vi "TX ADU.vi"(8 "error in (no error)":errorcluster, 9 "PDU_req in":T1={"Function Code"=1, "Data"=[], "RTU_DataBytes"=0}, 10 "VISA resource in":refnum<visa-resource-name>, 11 "MB_ADU in":refnum<class "MB_ADU_ASCII.lvclass">) -> (0 "error out":errorcluster, 1 "PDU_req out":T1={"Function Code"=1, "Data"=[], "RTU_DataBytes"=0}, 2 "VISA resource out":refnum<visa-resource-name>, 3 "MB_ADU out":refnum<class "MB_ADU_ASCII.lvclass">)   [LabVIEW 2012, in "MB Master.lvlib" / "MB_ADU_ASCII.lvclass"]
doc: "Defines the transmit procedure for a Modbus ASCII ADU. The PDU to be transmitted should be written to PDU_req prior to calling this VI."
uses:
  MB_ADU_ASCII.lvclass
  MB_PDU/MB_PDU_Cluster.ctl
  MB_ADU/MB_ADU.lvclass/MB_ADU.ctl
  MB_ADU/Read Slave ID.vi
  MB_ADU/Write TX Data.vi
  MB_ADU/Write TX Timestamp.vi
  MB Master.lvlib
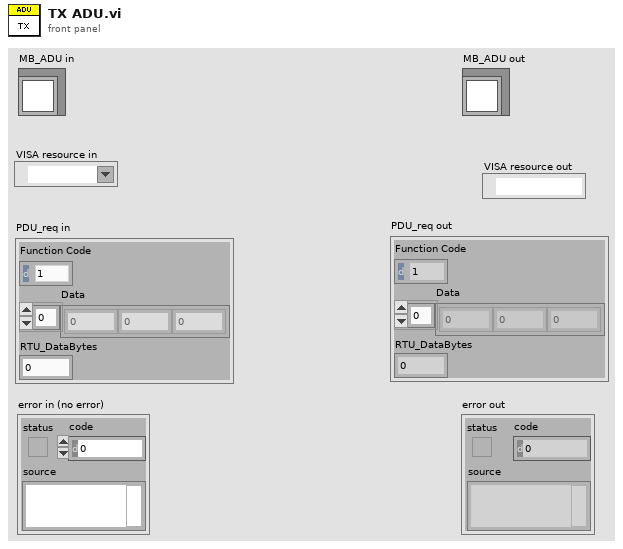
[diagram p1: front panel]
types:
  T1 = typedef "MB Master.lvlib/MB_PDU_Cluster.ctl" = cluster{"Function Code":u8, "Data":u8[], "RTU_DataBytes":i32}
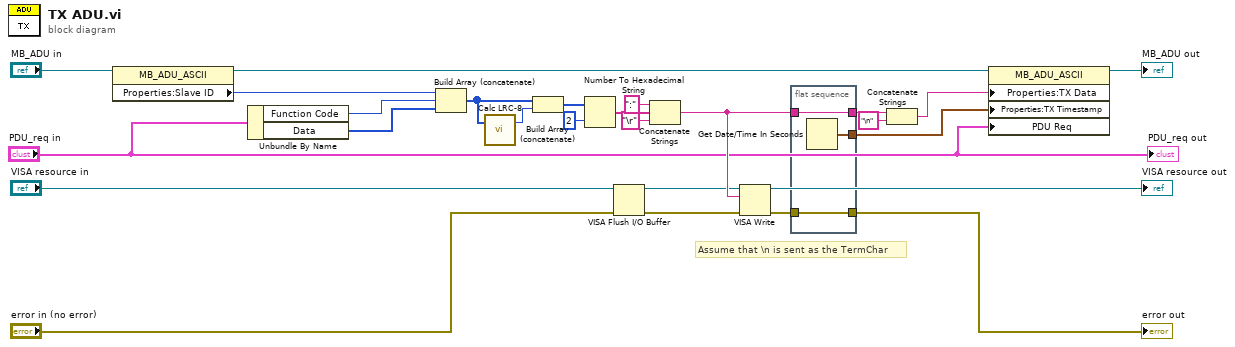
[diagram p0: block diagram]
diagram:
  # "Assume that \\n is sent as the TermChar"
  n1 = property class="MB_ADU_ASCII"(reference="MB_ADU in") -> (reference out=w11:refnum<class "MB_ADU_ASCII.lvclass">, "Properties:Slave ID"=w24:u8)  [unwired: 1 in, 1 out]
  n2 = Unbundle By Name("PDU_req in") -> ("Function Code"=w3:u8, "Data"=w2:u8[])
  n3 = Build Array (concatenate)(w24, w3, w2) -> (w23:u8[])
  n4 = call "Calc LRC-8.vi"("Frame in"=w23) -> ("LRC-8"=w22:u8)  [unwired: 2 in]
  n5 = Build Array (concatenate)(w23, w22) -> (w21:u8[])
  n6 = Number To Hexadecimal String(1:i16 2 ("width (-)"), 2:w21) -> (0:w19:string[])
  n7 = VISA Flush I/O Buffer(VISA resource name="VISA resource in", error in (no error)="error in (no error)") -> (VISA resource name out=w5:refnum<visa-resource-name>, error out=w4:errorcluster)  [unwired: 1 in]
  n8 = Concatenate Strings(":" ("string"), w19, "\r" ("string")) -> (w16:string)
  n9 = VISA Write(VISA resource name=w5, write buffer=w16, error in (no error)=w4) -> (VISA resource name out=→"VISA resource out":refnum<visa-resource-name>, error out=w9:errorcluster)  [unwired: 1 out]
  n10 = flat-sequence {
    tunnel: w16 -> [w29]
    tunnel: [w29] -> w15
    tunnel: [w28] -> w12
    tunnel: w9 -> [w27]
    tunnel: [w27] -> w8
    frame #0 {
      n11 = Get Date/Time In Seconds() -> (seconds since 1Jan1904=w28:timestamp)
    }
  }
  n12 = Concatenate Strings(w15, "\n" ("string")) -> (w13:string)
  n13 = property class="MB_ADU_ASCII"(reference=w11, "Properties:TX Data"=w13, "Properties:TX Timestamp"=w12, "PDU Req"="PDU_req in") -> (reference out=→"MB_ADU out":refnum<class "MB_ADU_ASCII.lvclass">)  [unwired: 1 in, 1 out]
  "error out" <- w8
  "PDU_req out" <- "PDU_req in"
